vi "GetQueuebyName.vi"(7 "Instance":i32, 8 "error in (no error)":errorcluster, 11 "Name":string) -> (0 "error out":errorcluster, 1 "Event?":bool, 2 "queue out":refnum<queue>)   [LabVIEW 2017, in "Communication.lvlib"]
uses:
  Communication.lvlib
  SubVIs/MsgData.ctl
  SubVIs/MsgAck.ctl
  SubVIs/QueueRepo.Action.ctl
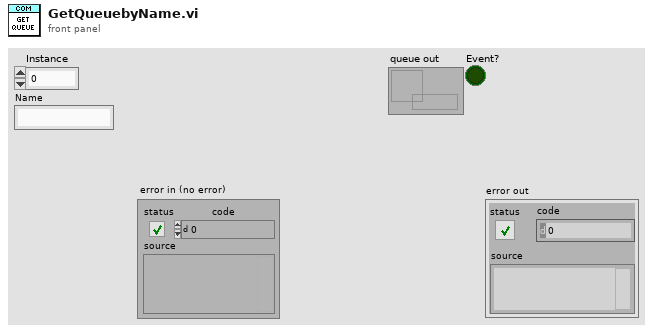
[diagram p1: front panel]
types:
  T1 = typedef "Communication.lvlib/QueueRepo.Action.ctl" = enum16{"Add", "Get", "Destroy", "Get All", "Clear"}
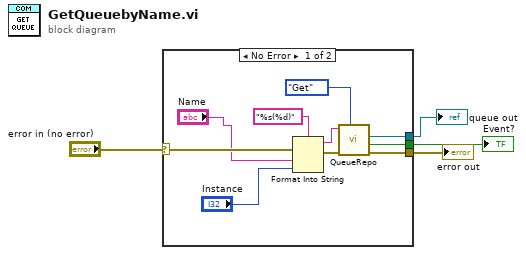
[diagram p0: block diagram]
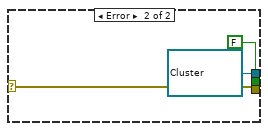
[diagram p2: hidden frame]
diagram:
  n1 = case shown="No Error" "error in (no error)" {
    selector: "error in (no error)" -> [w6 w17]
    tunnel: [w11 w17] -> w3
    tunnel: [w8 refnum<queue> refnum ("queue out")] -> w2
    tunnel: [w7 FALSE ("Event?")] -> w1
    frame No Error {
      n2 = Format Into String(format string="%s(%d)", error in=w6, "Name", "Instance") -> (resulting string=w10:string, error out=w12:errorcluster)  [unwired: 1 in]
      n3 = call "QueueRepo.vi"("Action"=QueueRepo.Action."Get", "error in (no error)"=w12, "Name"=w10) -> ("error out"=w11:errorcluster, "Event?"=w7:bool, "queue out"=w8:refnum<queue>)  [unwired: 5 in, 1 out]
    }
    frame Error {
    }
  }
  "error out" <- w3
  "queue out" <- w2
  "Event?" <- w1
